vi "Main.vi"() -> ()   [LabVIEW 2015]
doc: "The myRIO Project template acquires acceleration data from the onboard accelerometer and displays the changes of acceleration values in a waveform chart."
uses:
  <vilib>/myRIO/Instrument Drivers/Onboard IO/AI/typedefs/AI Reference.ctl
  <vilib>/myRIO/Common/Instrument Driver Framework/Utilities/typedefs/myRIO Generic Hardware Reference.ctl
  <vilib>/myRIO/Common/Instrument Driver Framework/Utilities/typedefs/Hardware Version Enum.ctl
  <vilib>/myRIO/Common/Instrument Driver Framework/Utilities/typedefs/myRIO v1.0 Reference.ctl
  <vilib>/myRIO/Common/Instrument Driver Framework/Utilities/typedefs/Generic FPGA Reference.ctl
  <vilib>/myRIO/Common/Instrument Driver Framework/myRIO v1.0/AI/typedefs/AI Channels List.ctl
  <vilib>/myRIO/Common/Instrument Driver Framework/myRIO v1.0/AI/typedefs/AI Channels Enum.ctl
  <vilib>/myRIO/Common/Instrument Driver Framework/Utilities/typedefs/Analog Scaling Constants List.ctl
  <vilib>/myRIO/Common/Instrument Driver Framework/Utilities/typedefs/Analog Scaling Constants.ctl
  <vilib>/userdefined/High Color/nirio_resource_hc.ctl
  <vilib>/myRIO/Instrument Drivers/Onboard IO/DIO/typedefs/DIO Reference.ctl
  <vilib>/myRIO/Common/Instrument Driver Framework/myRIO v1.0/DIO/typedefs/DIO Channels List.ctl
  <vilib>/myRIO/Common/Instrument Driver Framework/myRIO v1.0/DIO/typedefs/DIO Channels Enum.ctl
  <vilib>/myRIO/Instrument Drivers/Onboard IO/PWM/typedefs/PWM Reference.ctl
  <vilib>/myRIO/Common/Instrument Driver Framework/myRIO v1.0/PWM/typedefs/PWM Channels Enum.ctl
  <vilib>/myRIO/Instrument Drivers/Onboard IO/PWM/typedefs/PWM Configuration.ctl
  <vilib>/myRIO/Instrument Drivers/Onboard Devices/Accelerometer/typedefs/Accelerometer Reference.ctl
  <vilib>/myRIO/Common/Instrument Driver Framework/myRIO v1.0/Accelerometer/typedefs/Accelerometer Channels List.ctl
  <vilib>/myRIO/Common/Instrument Driver Framework/myRIO v1.0/Accelerometer/typedefs/Accelerometer Channels Enum.ctl
  <vilib>/myRIO/Common/Instrument Driver Framework/Utilities/vis/Is FPGA Ref Available.vi
  <vilib>/myRIO/Common/Instrument Driver Framework/myRIO v1.0/DIO/vis/myRIO v1.1 Open DIO.vi
  <vilib>/myRIO/Instrument Drivers/Onboard IO/DIO/vis/Read.vi
  <vilib>/myRIO/Common/Instrument Driver Framework/myRIO v1.0/AI/vis/myRIO v1.1 Open AI.vi
  <vilib>/myRIO/Instrument Drivers/Onboard IO/AI/vis/Read.vi
  <vilib>/myRIO/Instrument Drivers/Onboard IO/DIO/vis/Write.vi
  <vilib>/myRIO/Common/Instrument Driver Framework/myRIO v1.0/PWM/vis/myRIO v1.1 Open PWM.vi
  <vilib>/myRIO/Instrument Drivers/Onboard IO/PWM/vis/Set Duty Cycle and Frequency.vi
  <vilib>/myRIO/Common/Instrument Driver Framework/myRIO v1.0/Accelerometer/vis/myRIO v1.1 Open Accelerometer.vi
  <vilib>/myRIO/Instrument Drivers/Onboard Devices/Accelerometer/vis/Read.vi
  <vilib>/myRIO/Common/Instrument Driver Framework/Utilities/vis/Validate Channels.vi
  <vilib>/myRIO/Common/Instrument Driver Framework/myRIO v1.0/DIO/vis/myRIO v1.0 Reserve DIO.vi
  <vilib>/myRIO/Common/Instrument Driver Framework/myRIO v1.0/AI/vis/myRIO v1.0 Reserve AI.vi
  <vilib>/myRIO/Common/Instrument Driver Framework/myRIO v1.0/PWM/vis/myRIO v1.0 Reserve PWM.vi
  <vilib>/myRIO/Common/Instrument Driver Framework/myRIO v1.0/Accelerometer/vis/myRIO v1.0 Reserve Accelerometer.vi
  <vilib>/myRIO/Common/Instrument Driver Framework/myRIO v1.0/UART/vis/myRIO v1.0 Close UART.vi
  <vilib>/myRIO/Common/Instrument Driver Framework/myRIO v1.0/Resource Manager/vis/myRIO v1.0 Reserve Channel List.vi
  <vilib>/myRIO/Common/Instrument Driver Framework/myRIO v1.0/DIO/vis/myRIO v1.0 Build MUX Configuration DIO.vi
  <vilib>/myRIO/Common/Instrument Driver Framework/myRIO v1.0/AI/vis/myRIO v1.0 Build MUX Configuration AI.vi
  <vilib>/myRIO/Common/Instrument Driver Framework/myRIO v1.0/PWM/vis/myRIO v1.0 Build MUX Configuration PWM.vi
  <vilib>/myRIO/Common/Instrument Driver Framework/myRIO v1.0/Accelerometer/vis/myRIO v1.0 Build MUX Configuration Accelerometer.vi
  <vilib>/myRIO/Common/Instrument Driver Framework/myRIO v1.0/Resource Manager/vis/myRIO v1.0 Reserve Channel.vi
  <vilib>/myRIO/Common/Instrument Driver Framework/myRIO v1.0/Resource Manager/vis/myRIO v1.0 Unreserve Channel.vi
  <vilib>/myRIO/Common/Instrument Driver Framework/myRIO v1.0/Resource Manager/vis/myRIO v1.0 Create Configuration List.vi
  <vilib>/myRIO/Common/Instrument Driver Framework/myRIO v1.0/Resource Manager/vis/myRIO v1.0 Build Mutex Name.vi
  <vilib>/Utility/VariantDataType/GetNumericInfo.vi
  <vilib>/Utility/error.llb/Error Cluster From Error Code.vi
  <vilib>/myRIO/Common/Instrument Driver Framework/myRIO v1.0/myRIO v1.1 Open.vi
  <vilib>/myRIO/Common/Instrument Driver Framework/myRIO v1.0/AI/vis/myRIO v1.0 Get Scaling Constants AI.vi
  <vilib>/myRIO/Common/Instrument Driver Framework/Utilities/vis/IO Manager.vi
  <vilib>/myRIO/Common/Instrument Driver Framework/Utilities/vis/Configuration Manager.vi
  <vilib>/myRIO/Common/Instrument Driver Framework/myRIO v1.0/myRIO v1.0 Close.vi
  <vilib>/myRIO/Common/Instrument Driver Framework/myRIO v1.0/AI/vis/myRIO v1.0 Read AI.vi
  <vilib>/addons/control/pid/pid.llb/PID (DBL).vi
  <vilib>/myRIO/Common/Instrument Driver Framework/myRIO v1.0/Resource Manager/vis/myRIO v1.0 Configure IO.vi
  <vilib>/myRIO/Common/Instrument Driver Framework/myRIO v1.0/DIO/vis/myRIO v1.0 Read DIO.vi
  <vilib>/myRIO/Common/Instrument Driver Framework/myRIO v1.0/PWM/vis/myRIO v1.0 Write PWM.vi
  <vilib>/myRIO/Common/Instrument Driver Framework/myRIO v1.0/DIO/vis/myRIO v1.0 Write DIO.vi
  <vilib>/myRIO/Common/Instrument Driver Framework/myRIO v1.0/Accelerometer/vis/myRIO v1.0 Get Scaling Constant Accelerometer.vi
  <vilib>/myRIO/Common/Instrument Driver Framework/myRIO v1.0/Accelerometer/vis/myRIO v1.0 Read Accelerometer.vi
  <vilib>/myRIO/Common/Instrument Driver Framework/Utilities/vis/FPGA Ref Manager.vi
  <vilib>/myRIO/Common/Instrument Driver Framework/myRIO v1.0/myRIO v1.0 Reset FPGA.vi
  <vilib>/myRIO/Common/Instrument Driver Framework/myRIO v1.0/IRQ/vis/myRIO v1.0 IRQ Info FGV.vi
  <vilib>/myRIO/Common/Instrument Driver Framework/myRIO v1.0/IRQ/vis/myRIO v1.0 Timer IRQ Info FGV.vi
  <vilib>/myRIO/Common/Instrument Driver Framework/myRIO v1.0/IRQ/vis/myRIO v1.0 ISR Agent.vi
  <vilib>/myRIO/Express VI/Onboard IO/AI/AI Express VI.xnode
  <vilib>/myRIO/Instrument Drivers/Onboard IO/AI/vis/myRIO AI Open.xnode
  <vilib>/myRIO/Express VI/Onboard IO/DI/DI Express VI.xnode
  <vilib>/myRIO/Instrument Drivers/Onboard IO/DIO/vis/myRIO DIO Open.xnode
  <vilib>/myRIO/Express VI/Onboard IO/PWM/PWM Express VI.xnode
  <vilib>/myRIO/Instrument Drivers/Onboard IO/PWM/vis/myRIO PWM Open.xnode
  <vilib>/myRIO/Express VI/Onboard IO/DO/DO Express VI.xnode
  <vilib>/myRIO/Express VI/Onboard Devices/Accelerometer/Accelerometer Express VI.xnode
  <vilib>/myRIO/Instrument Drivers/Onboard Devices/Accelerometer/vis/myRIO Accelerometer Open.xnode
  <vilib>/myRIO/Instrument Drivers/Utilities/Utilities.lvlib
  <vilib>/myRIO/Instrument Drivers/Onboard Devices/Accelerometer/Accelerometer.lvlib
  <vilib>/myRIO/Instrument Drivers/Onboard IO/PWM/PWM.lvlib
  <vilib>/myRIO/Instrument Drivers/Onboard IO/DIO/DIO.lvlib
  <vilib>/myRIO/Instrument Drivers/Onboard IO/AI/AI.lvlib
  <vilib>/addons/control/pid/NI_PID_pid.lvlib
panel:
  out "波形图表 2":dbl(graph)
  out "波形图表":dbl(graph)
  out "数值 3":dbl
  out "数值 2":dbl
  out "数值":dbl
  in  "PID gains":T1={"proportional gain (Kc)"=1.0, "integral time (Ti, min)"=0.01, "derivative time (Td, min)"=0.0} caption="PID增益" {"derivative time (Td, min)" format="%.3f"; "integral time (Ti, min)" format="%.3f"; "proportional gain (Kc)" format="%.3f"}
  out "Acceleration":T2(graph)
  out "error out":errorcluster
  in  "Stop":bool
  # "Overview: The myRIO Project template acquires acceleration data from the onboard accelerometer and displays the changes of acceleration values in a waveform chart.\nInstructions:\n1. Check the myRIO target IP address in the project and make sure the target IP address is correct. \n2. Run this VI."
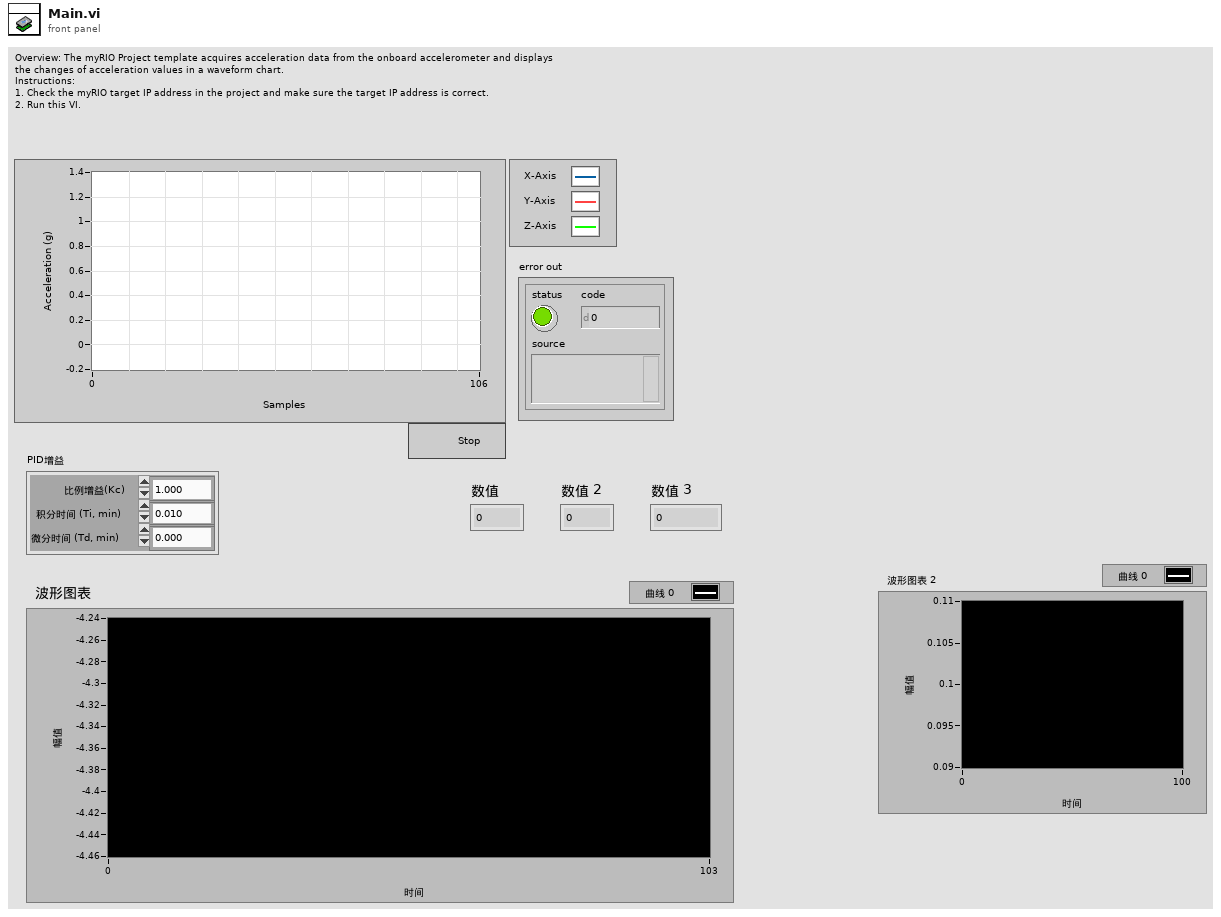
[diagram p1: front panel]
types:
  T1 = cluster{"proportional gain (Kc)":dbl, "integral time (Ti, min)":dbl, "derivative time (Td, min)":dbl}
  T2 = cluster{"X-Axis":dbl, "Y-Axis":dbl, "Z-Axis":dbl}
  T3 = typedef "DIO.lvlib/DIO Reference.ctl" = cluster{"myRIO Reference":T4, "DIO Channels List":T8}
  T4 = typedef "myRIO Generic Hardware Reference.ctl" = cluster{"myRIO Model":T5, "myRIO Hardware Reference":T6}
  T5 = typedef "Hardware Version Enum.ctl" = enum16{"Unknown", "myRIO-1900", "myRIO-1950", "roboRIO"}
  T6 = typedef "myRIO v1.0 Reference.ctl" = cluster{"Generic FPGA Reference":T7, "Allow multiple opens":bool}
  T7 = typedef "Generic FPGA Reference.ctl" = refnum<k20>
  T8 = typedef "DIO Channels List.ctl" = T9[]
  T9 = typedef "DIO Channels Enum.ctl" = enum16{"Not Connected", "C/DIO0", "C/DIO1", "C/DIO2", "C/DIO3", "C/DIO4", "C/DIO5", "C/DIO6", "C/DIO7", "A/DIO0", "A/DIO1", "A/DIO2", "A/DIO3", "A/DIO4", "A/DIO5", "A/DIO6", "A/DIO7", "A/DIO8", "A/DIO9", "A/DIO10", "A/DIO11", "A/DIO12", "A/DIO13", "A/DIO14", "A/DIO15", "B/DIO0", "B/DIO1", "B/DIO2", "B/DIO3", "B/DIO4", "B/DIO5", "B/DIO6", "B/DIO7", "B/DIO8", "B/DIO9", "B/DIO10", "B/DIO11", "B/DIO12", "B/DIO13", "B/DIO14", "B/DIO15", "LED0", "LED1", "LED2", "LED3", "Button0", "DIO/DIO0", "DIO/DIO1", "DIO/DIO2", "DIO/DIO3", "DIO/DIO4", "DIO/DIO5", "DIO/DIO6", "DIO/DIO7", "DIO/DIO8", "DIO/DIO9", "SPI/CS0", "SPI/CS1", "SPI/CS2", "SPI/CS3", "LED RADIO (Green)", "LED RADIO (Red)", "LED COMM (Green)", "LED COMM (Red)", "LED MODE (Green)", "LED MODE (Red)"}
  T10 = typedef "nirio_resource_hc.ctl" = tag
  T11 = typedef "AI.lvlib/AI Reference.ctl" = cluster{"myRIO Reference":T4, "AI Channels List":T12, "AI Scaling Constants List":T14}
  T12 = typedef "AI Channels List.ctl" = T13[]
  T13 = typedef "AI Channels Enum.ctl" = enum16{"Not Connected", "AudioIn/Left", "AudioIn/Right", "C/AI0", "C/AI1", "A/AI0", "A/AI1", "A/AI2", "A/AI3", "B/AI0", "B/AI1", "B/AI2", "B/AI3", "AI/AI0", "AI/AI1", "AI/AI2", "AI/AI3"}
  T14 = typedef "Analog Scaling Constants List.ctl" = T15[]
  T15 = typedef "Analog Scaling Constants.ctl" = cluster{"LSB Weight (Volts)":dbl, "Offset (Volts)":dbl, "Signed?":bool}
  T16 = typedef "PWM.lvlib/PWM Reference.ctl" = cluster{"myRIO Reference":T4, "PWM Channels Enum":T17, "PWM Configuration":T18}
  T17 = typedef "PWM Channels Enum.ctl" = enum16{"Not Connected", "C/PWM0", "C/PWM1", "A/PWM0", "A/PWM1", "A/PWM2", "B/PWM0", "B/PWM1", "B/PWM2", "PWM/PWM0", "PWM/PWM1", "PWM/PWM2", "PWM/PWM3", "PWM/PWM4", "PWM/PWM5", "PWM/PWM6", "PWM/PWM7", "PWM/PWM8", "PWM/PWM9"}
  T18 = typedef "PWM.lvlib/PWM Configuration.ctl" = cluster{"Frequency":dbl, "Duty Cycle":dbl}
  T19 = typedef "Accelerometer.lvlib/Accelerometer Reference.ctl" = cluster{"myRIO Reference":T4, "Accelerometer Channels List":T20, "LSB Weight":dbl}
  T20 = typedef "Accelerometer Channels List.ctl" = T21[]
  T21 = typedef "Accelerometer Channels Enum.ctl" = enum16{"Not Connected", "X-Axis", "Y-Axis", "Z-Axis"}
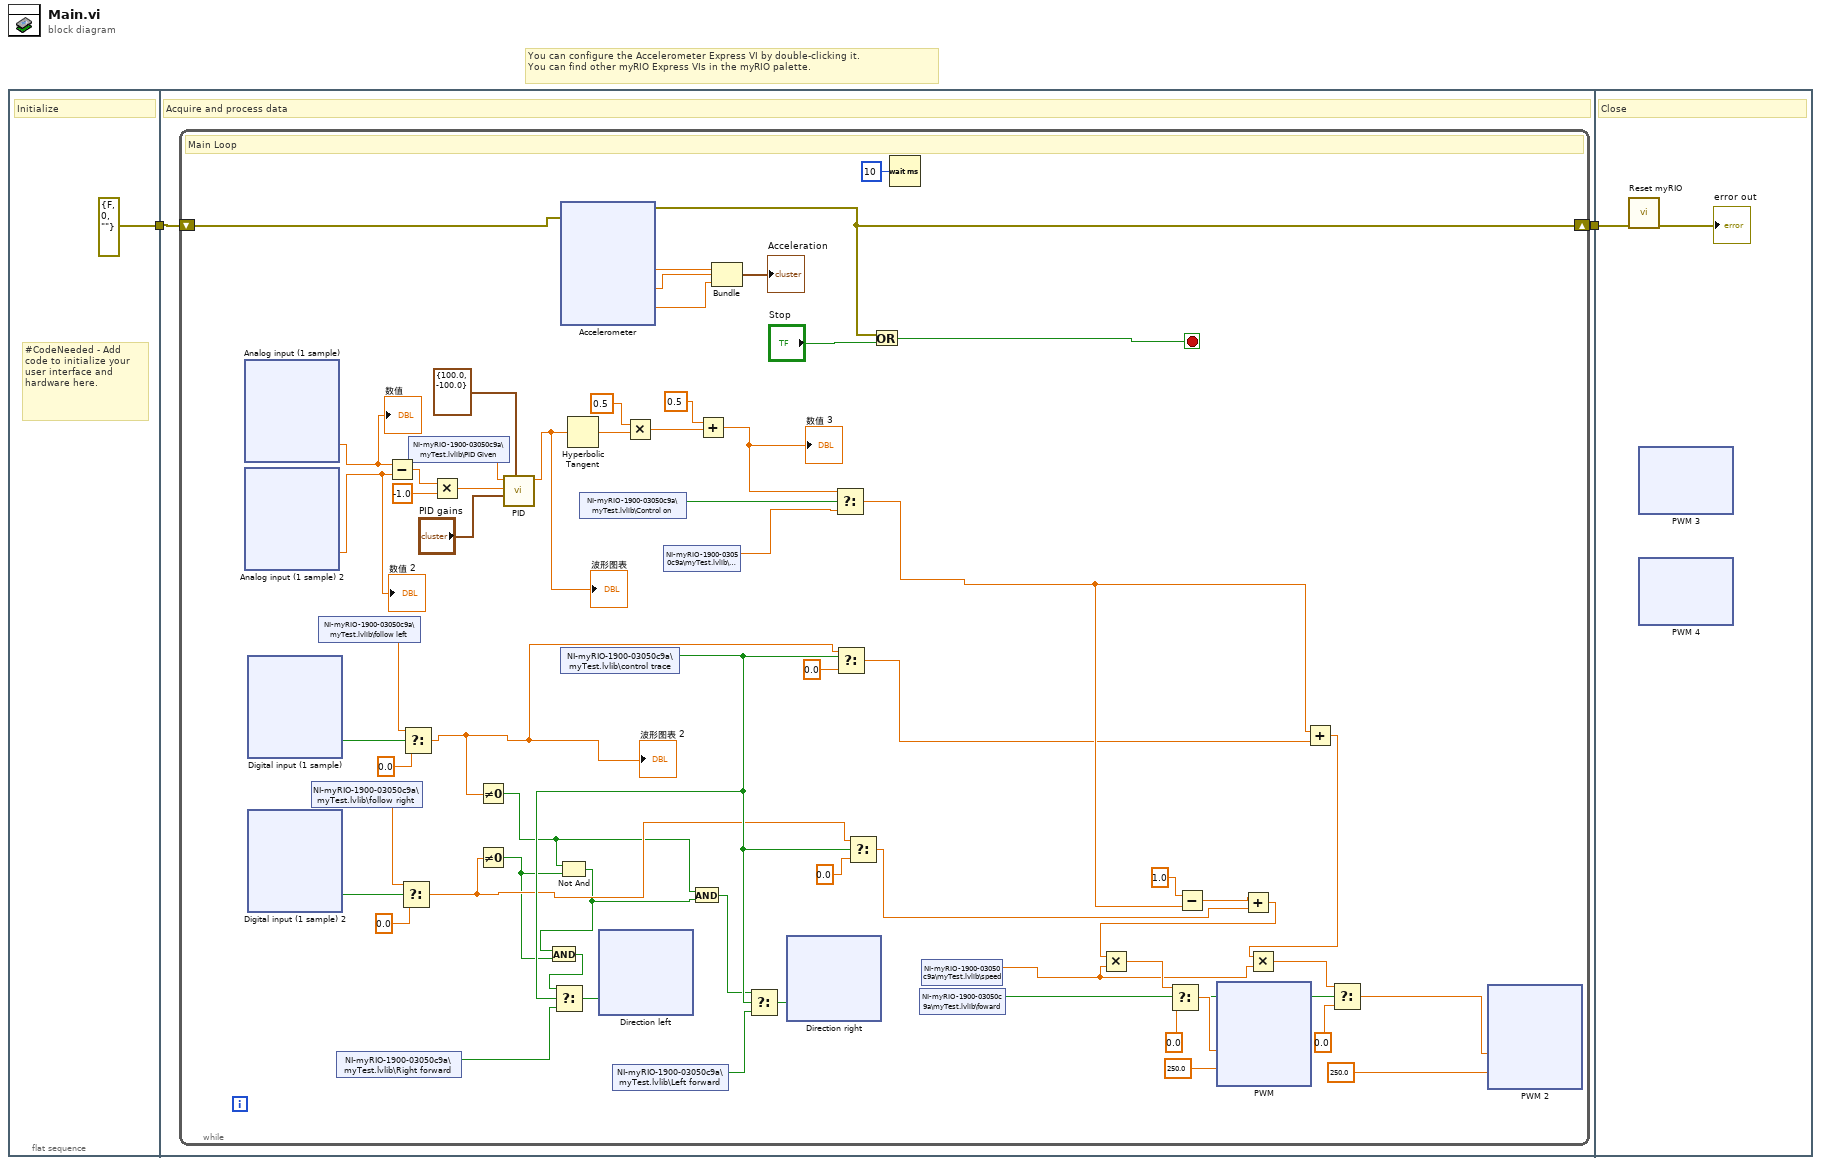
[diagram p0: block diagram]
diagram:
  # "You can configure the Accelerometer Express VI by double-clicking it.\nYou can find other myRIO Express VIs in the myRIO palette."
  n1 = flat-sequence {
    tunnel: [errorcluster {"status"=FALSE, "code"=0, "source"=""} ("error in (no error)")] -> w2
    tunnel: w2 -> [w5]
    tunnel: [w4] -> w1
    tunnel: w1 -> [w392]
    frame #0 {
      # "#CodeNeeded - Add code to initialize your user interface and hardware here."
      # "Initialize"
    }
    frame #1 {
      # "Acquire and process data"
      n2 = while {
        shift-right: [w63] -> w4
        shift-left: w5 -> [w59]
        stop <- w66 stop-if-true
        # "Main Loop"
        n3 = xnode "Analog input (1 sample)"() -> ("A/AI2 (Pin 7)"=w42:dbl)  [unwired: 1 in, 1 out]
        "数值" <- w42
        n4 = xnode "Analog input (1 sample) 2"() -> ("A/AI1 (Pin 5)"=w43:dbl)  [unwired: 1 in, 1 out]
        "数值 2" <- w43
        n5 = xnode "Digital input (1 sample)"() -> ("A/DIO1 (Pin 13)"=w22:bool)  [unwired: 1 in, 1 out]
        n6 = xnode "Digital input (1 sample) 2"() -> ("A/DIO0 (Pin 11)"=w23:bool)  [unwired: 1 in, 1 out]
        n7 = shared-variable "NI-myRIO-1900-03050c9a\\myTest.lvlib\\follow right"() -> (w19:dbl)  [unwired: 1 in, 1 out]
        n8 = shared-variable "NI-myRIO-1900-03050c9a\\myTest.lvlib\\follow left"() -> (w20:dbl)  [unwired: 1 in, 1 out]
        n9 = shared-variable "NI-myRIO-1900-03050c9a\\myTest.lvlib\\Right forward"() -> (w18:bool)  [unwired: 1 in, 1 out]
        n10 = Subtract(x=w42, y=w43) -> (x-y=w35:dbl)
        n11 = Select(t=w19, s=w23, f=0.0 ("x")) -> (s? t:f=w13:dbl)
        n12 = Select(t=w20, s=w22, f=0.0 ("x")) -> (s? t:f=w12:dbl)
        "波形图表 2" <- w12
        n13 = shared-variable "NI-myRIO-1900-03050c9a\\myTest.lvlib\\PID Given"() -> (w36:dbl)  [unwired: 1 in, 1 out]
        n14 = Multiply(x=w35, y=-1.0) -> (x*y=w33:dbl)
        n15 = Not Equal To 0?(x=w12) -> (x != 0?=w9:bool)
        n16 = Not Equal To 0?(x=w13) -> (x != 0?=w11:bool)
        n17 = call-poly <vilib>:"PID.vi"("output range"=cluster{"output high":dbl, "output low":dbl} {"output high"=100.0, "output low"=-100.0}, "PID gains"="PID gains", "process variable"=w33, "setpoint"=w36) -> ("output"=w37:dbl)  [unwired: 6 in, 1 out]
        "波形图表" <- w37
        n18 = Not And(1:w11, 2:w9) -> (0:w8:bool)
        n19 = And(x=w8, y=w11) -> (x .and. y?=w10:bool)
        n20 = xnode "Accelerometer"("error in (no error)"=w59) -> ("X-Axis"=w61:dbl, "Y-Axis"=w60:dbl, "Z-Axis"=w62:dbl, "error out"=w63:errorcluster)
        n21 = shared-variable "NI-myRIO-1900-03050c9a\\myTest.lvlib\\control trace"() -> (w14:bool)  [unwired: 1 in, 1 out]
        n22 = Select(t=w10, s=w14, f=w18) -> (s? t:f=w17:bool)
        n23 = Hyperbolic Tangent(1:w37) -> (0:w40:dbl)
        n24 = shared-variable "NI-myRIO-1900-03050c9a\\myTest.lvlib\\Control on"() -> (w45:bool)  [unwired: 1 in, 1 out]
        n25 = xnode "Direction left"("B/DIO3 (Pin 17)"=w17) -> ()  [unwired: 1 in, 1 out]
        n26 = shared-variable "NI-myRIO-1900-03050c9a\\myTest.lvlib\\Left forward"() -> (w15:bool)  [unwired: 1 in, 1 out]
        n27 = Multiply(x=0.5, y=w40) -> (x*y=w38:dbl)
        n28 = shared-variable "NI-myRIO-1900-03050c9a\\myTest.lvlib\\angle"() -> (w44:dbl)  [unwired: 1 in, 1 out]
        n29 = And(x=w9, y=w8) -> (x .and. y?=w7:bool)
        n30 = Add(x=0.5, y=w38) -> (x+y=w41:dbl)
        "数值 3" <- w41
        n31 = Bundle("X-Axis"=w61, "Y-Axis"=w60, "Z-Axis"=w62) -> (→"Acceleration":T2)  [unwired: 1 in]
        n32 = Select(t=w7, s=w14, f=w15) -> (s? t:f=w16:bool)
        n33 = xnode "Direction right"("A/DIO3 (Pin 17)"=w16) -> ()  [unwired: 1 in, 1 out]
        n34 = Select(t=w41, s=w45, f=w44) -> (s? t:f=w26:dbl)
        n35 = Select(t=w12, s=w14, f=0.0) -> (s? t:f=w25:dbl)
        n36 = Select(t=w13, s=w14, f=0.0) -> (s? t:f=w24:dbl)
        n37 = Or(x=w63, y="Stop") -> (x .or. y?=w66:bool)
        n38 = Wait (ms)(milliseconds to wait=u32 10) -> ()  [unwired: 1 out]
        n39 = shared-variable "NI-myRIO-1900-03050c9a\\myTest.lvlib\\foward"() -> (w52:bool)  [unwired: 1 in, 1 out]
        n40 = shared-variable "NI-myRIO-1900-03050c9a\\myTest.lvlib\\speed"() -> (w32:dbl)  [unwired: 1 in, 1 out]
        n41 = Subtract(x=1.0, y=w26) -> (x-y=w28:dbl)
        n42 = Add(x=w28, y=w24) -> (x+y=w27:dbl)
        n43 = Multiply(x=w27, y=w32) -> (x*y=w50:dbl)
        n44 = Select(t=w50, s=w52, f=0.0) -> (s? t:f=w53:dbl)
        n45 = xnode "PWM"("Duty Cycle"=w53, "Frequency [Hz]"=250.0) -> ()  [unwired: 1 in, 1 out]
        n46 = Add(x=w26, y=w25) -> (x+y=w29:dbl)
        n47 = Multiply(x=w29, y=w32) -> (x*y=w49:dbl)
        n48 = Select(t=w49, s=w52, f=0.0) -> (s? t:f=w54:dbl)
        n49 = xnode "PWM 2"("Duty Cycle"=w54, "Frequency [Hz]"=250.0) -> ()  [unwired: 1 in, 1 out]
      }
    }
    frame #2 {
      # "Close"
      n50 = call <vilib>:"Reset myRIO.vi"("error in (no error)"=w392) -> ("error out"=→"error out":errorcluster)  [unwired: 10 in]
      n51 = xnode "PWM 3"() -> ()  [unwired: 1 in, 1 out]
      n52 = xnode "PWM 4"() -> ()  [unwired: 1 in, 1 out]
    }
  }
